vi "Update Popup Image Window Image.vi"(8 "error in (no error)":errorcluster, 10 "Image":T1, 11 "UI in":refnum<class "UI.lvclass">) -> (0 "error out":errorcluster)   [LabVIEW 2020, in "AR Example.lvlib" / "UI.lvclass"]
uses:
  UI.lvclass
  UI.lvclass/UI.ctl
  g_ar_toolkit.image/ARGB Image.ctl
  g_ar_toolkit.image/g_ar_toolkit.image.lvlib
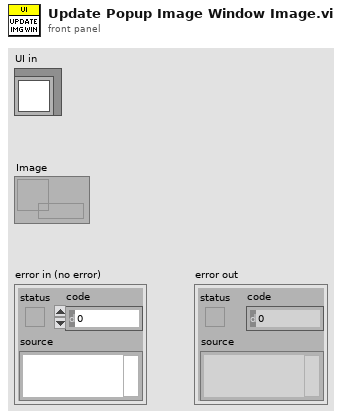
[diagram p1: front panel]
types:
  T1 = typedef "g_ar_toolkit.image.lvlib/ARGB Image.ctl" = refnum<data-value>
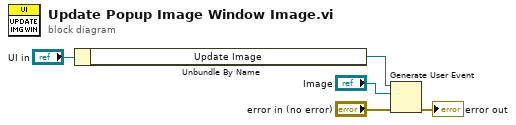
[diagram p0: block diagram]
diagram:
  n1 = Unbundle By Name("UI in") -> ("Update Image"=w4:refnum<user-event>)
  n2 = Generate User Event(user event=w4, event data cluster="Image", error in="error in (no error)") -> (error out=→"error out":errorcluster)  [unwired: 1 in, 1 out]
